vi "RSZVB Import Trace as Limit Line.vi"(5 "Stimulus Offset (0.0 Hz)":dbl format="%^.3e", 6 "Trace Name (Trc1)":string="Trc1", 7 "Response Offset (0.0 dB)":dbl format="%^.3e", 8 "error in (no error)":errorcluster {"code" format="%.0x"}, 9 "Limit Line Type (2: Upper)":i32(ring)=2 items=["Lower"=2, "Upper"=1], 10 "Channel (Trace) (1)":i32=1, 11 "VISA session":refnum<visa-resource-name>) -> (0 "error out":errorcluster {"code" format="%.0x"}, 3 "dup VISA session":refnum<visa-resource-name>)   [LabVIEW 2011]
doc: "This VI generates an lower (upper) limit line using the stimulus values of a data or memory trace and specified offset values.\n\nRemote-control command(s):\nCALCulate<Ch/Tr>:LIMit:LOWer:FEED <stimulus_offset>,<response_offset>[,<trace_name>]\nCALCulate<Ch/Tr>:LIMit:UPPer:FEED <stimulus_offset>,<response_offset>[,<trace_name>]"
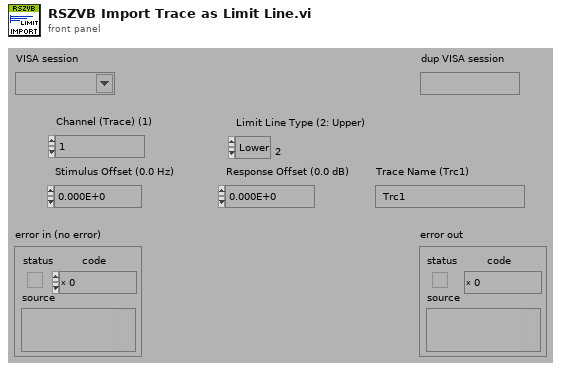
[diagram p1: front panel]
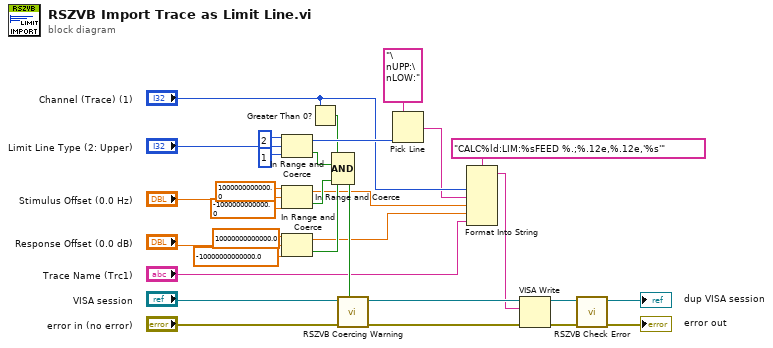
[diagram p0: block diagram]
diagram:
  n1 = In Range and Coerce(upper limit=2, x="Limit Line Type (2: Upper)", lower limit=1) -> (coerced(x)=w20:i32, In Range?=w24:bool)
  n2 = In Range and Coerce(upper limit=1000000000000.0, x="Stimulus Offset (0.0 Hz)", lower limit=-1000000000000.0 ("upper limit")) -> (coerced(x)=w3:dbl, In Range?=w7:bool)
  n3 = In Range and Coerce(upper limit=10000000000000.0, x="Response Offset (0.0 dB)", lower limit=-10000000000000.0 ("upper limit")) -> (coerced(x)=w2:dbl, In Range?=w4:bool)
  n4 = Greater Than 0?(x="Channel (Trace) (1)") -> (x > 0?=w19:bool)
  n5 = Compound Arithmetic op=AND(w19, w24, w7, w4) -> (w23:bool)
  n6 = call "RSZVB Coercing Warning.vi"("In Range?"=w23, "error in (no error)"="error in (no error)", "VISA session"="VISA session") -> ("error out"=w30:errorcluster, "dup VISA session"=w31:refnum<visa-resource-name>)  [unwired: 7 in]
  n7 = Pick Line(multi-line string="\nUPP:\nLOW:", line index=w20) -> (output string=w12:string)  [unwired: 1 in]
  n8 = Format Into String(format string="CALC%ld:LIM:%sFEED %.;%.12e,%.12e,'%s'", "Channel (Trace) (1)", w12, w3, w2, "Trace Name (Trc1)") -> (resulting string=w22:string)  [unwired: 2 in, 1 out]
  n9 = VISA Write(VISA resource name=w31, write buffer=w22, error in (no error)=w30) -> (VISA resource name out=w28:refnum<visa-resource-name>, error out=w29:errorcluster)  [unwired: 1 out]
  n10 = call "RSZVB Check Error.vi"("error in (no error)"=w29, "VISA session"=w28) -> ("error out"=→"error out":errorcluster, "dup VISA session"=→"dup VISA session":refnum<visa-resource-name>)  [unwired: 8 in]
